vi "多列列表框-单元格高亮效果.vi"(6 "活动单元格":T1 caption="活动单元格:活动单元格" {"Row" min=0}, 7 "动作（选中）":enum16{"选中", "不选"}(ring), 8 "错误输入（无错误）":errorcluster, 11 "引用":refnum<vi>) -> (0 "错误输出":errorcluster, 3 "引用输出":refnum<vi>)   [LabVIEW 2017]
doc: "保留列首单元格属性，整表单元格回复默认，然后更新单元格选中状态，并使之位置可见。"
uses:
  <vilib>/Utility/miscctls.llb/LVRowAndColumnTypeDef.ctl
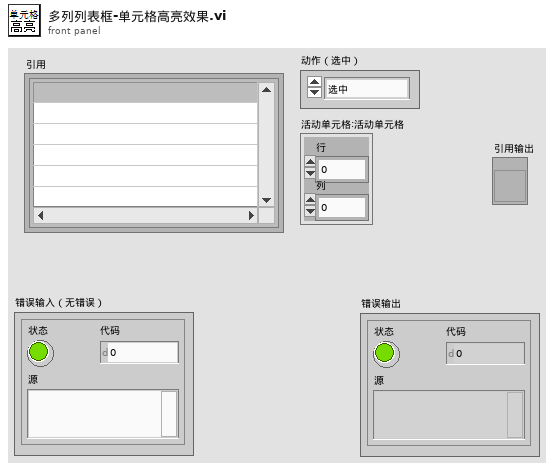
[diagram p1: front panel]
types:
  T1 = typedef "LVRowAndColumnTypeDef.ctl" = cluster{"Row":i32, "Column":i32}
  T2 = typedef "LVFontTypeDef.ctl" = cluster{"Font Name":string, "Size":u16, "Bold":bool, "Italic":bool, "Underline":bool, "Strikeout":bool, "Color":u32}
  T3 = typedef "LVRowAndColumnUnsignedTypeDef.ctl" = cluster{"Row":u32, "Column":u32}
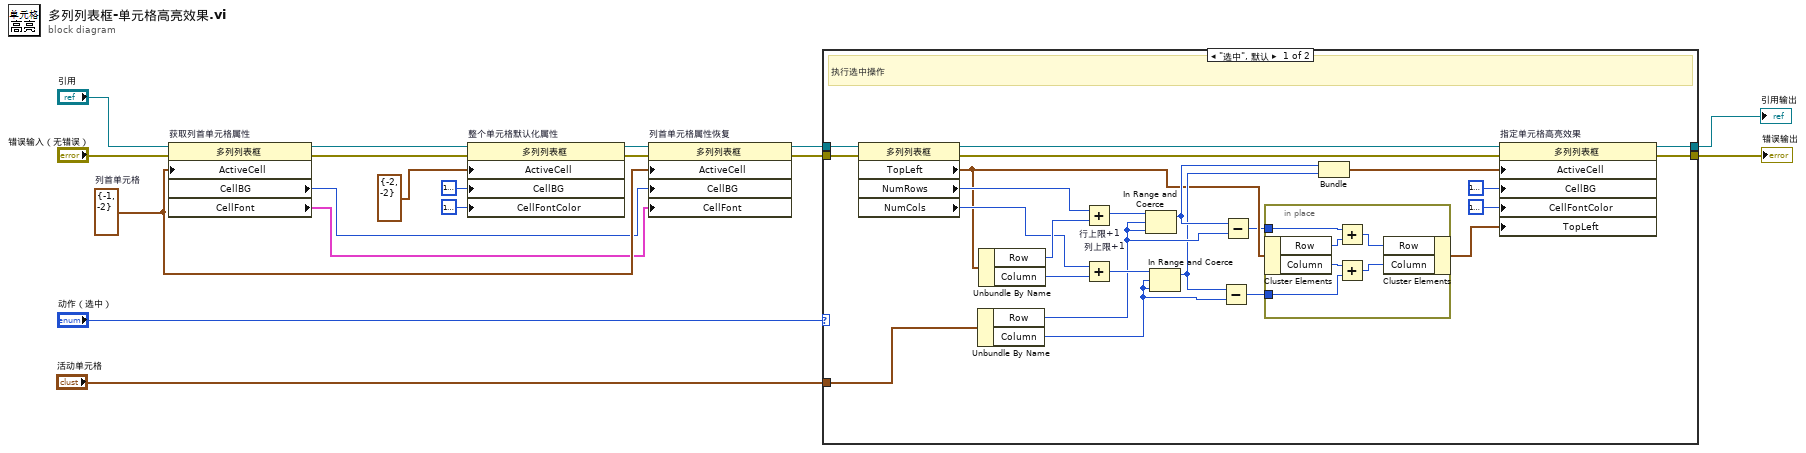
[diagram p0: block diagram]
diagram:
  w12 = T1 {"Row"=-1, "Column"=-2}  # 列首单元格
  n1 = property on="获取列首单元格属性" class="多列列表框"(reference="引用", error in="错误输入（无错误）", "ActiveCell"=w12) -> (reference out=w14:refnum<vi>, error out=w9:errorcluster, "CellBG"=w11:u32, "CellFont"=w10:T2)
  n2 = property on="整个单元格默认化属性" class="多列列表框"(reference=w14, error in=w9, "ActiveCell"=T1 {"Row"=-2, "Column"=-2} ("活动单元格:活动单元格"), "CellBG"=u32 16777226, "CellFontColor"=u32 16777222) -> (reference out=w13:refnum<vi>, error out=w8:errorcluster)
  n3 = property on="列首单元格属性恢复" class="多列列表框"(reference=w13, error in=w8, "ActiveCell"=w12, "CellBG"=w11, "CellFont"=w10) -> (reference out=w4:refnum<vi>, error out=w3:errorcluster)
  n4 = case shown="\"选中\", 默认" "动作（选中）" {
    tunnel: [w40 w49] -> w6
    tunnel: [w39 w50] -> w5
    tunnel: w4 -> [w38 w50]
    tunnel: w3 -> [w37 w49]
    tunnel: "活动单元格" -> [w34 _]
    frame "选中", Default {
      # "执行选中操作"
      n5 = property class="多列列表框"(reference=w38, error in=w37) -> (reference out=w36:refnum<vi>, error out=w35:errorcluster, "TopLeft"=w22:T3, "NumRows"=w31:u32, "NumCols"=w30:u32)
      n6 = Unbundle By Name(w34) -> ("Row"=w25:i32, "Column"=w23:i32)
      n7 = Unbundle By Name(w22) -> ("Row"=w33:u32, "Column"=w32:u32)
      n8 = Add "行上限+1"(x=w31, y=w33) -> (x+y=w29:u32)
      n9 = Add "列上限+1"(x=w30, y=w32) -> (x+y=w28:u32)
      n10 = In Range and Coerce(upper limit=w29, x=w25, lower limit=w25) -> (coerced(x)=w26:u32)  [unwired: 1 out]
      n11 = In Range and Coerce(upper limit=w28, x=w23, lower limit=w23) -> (coerced(x)=w24:u32)  [unwired: 1 out]
      n12 = Subtract(x=w24, y=w23) -> (x-y=w20:u32)
      n13 = Subtract(x=w26, y=w25) -> (x-y=w21:u32)
      n14 = in-place {
        in-place-border: w21 -> [w46]
        in-place-border: w20 -> [w45]
        n15 = in-place-cluster #1(w22) -> ("Row"=w48:u32, "Column"=w47:u32)
        n16 = Add(x=w46, y=w48) -> (x+y=w44:u32)
        n17 = Add(x=w47, y=w45) -> (x+y=w43:u32)
        n18 = in-place-cluster #1("Row"=w44, "Column"=w43) -> (w19:T3)
      }
      n19 = Bundle("Row"=w26, "Column"=w24) -> (w27:cluster{"Row":u32, "Column":u32})  [unwired: 1 in]
      n20 = property on="指定单元格高亮效果" class="多列列表框"(reference=w36, error in=w35, "ActiveCell"=w27, "CellBG"=u32 16777224, "CellFontColor"=u32 16777225, "TopLeft"=w19) -> (reference out=w39:refnum<vi>, error out=w40:errorcluster)
    }
    frame "不选" {
      # "不选单元格，全表格默认状态"
    }
  }
  "错误输出" <- w6
  "引用输出" <- w5
